vi "UI_Stop.vi"(0 "reference in":refnum<class "GUI.lvclass">, 5 "timeout ms":i32=1000, 11 "error in (no error)":errorcluster) -> (4 "reference out":refnum<class "GUI.lvclass">, 6 "timeout":bool, 10 "time":i32, 15 "error out":errorcluster)   [LabVIEW 2019, in "GUI.lvclass"]
uses:
  GUI.lvclass
  GUI.lvclass/GUI.ctl
  WindowsState.ctl
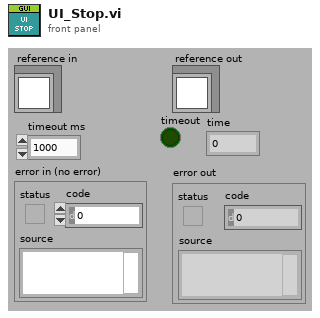
[diagram p1: front panel]
types:
  T1 = typedef "GUI.lvclass/WindowsState.ctl" = enum16{"NotReady", "Ready", "Inserted", "Opened"}
  T2 = typedef "GUI.lvclass/Shered Data.ctl" = cluster{"WindowsState":T1, "UI VI":refnum<vi>, "SubPnl":refnum<vi>}
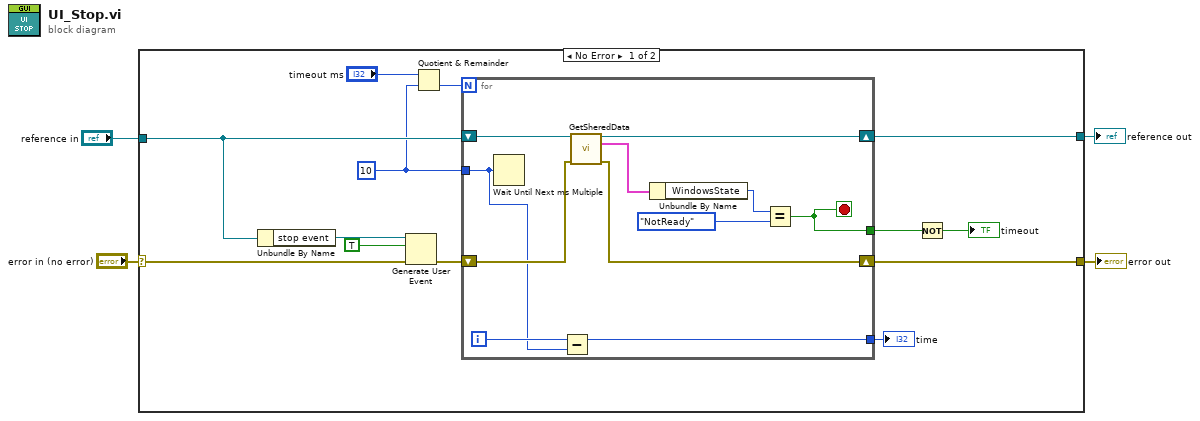
[diagram p0: block diagram]
diagram:
  n1 = case shown="No Error" "error in (no error)" {
    selector: "error in (no error)" -> [w17 w30]
    tunnel: [w10 w30] -> w3
    tunnel: [w11 w29] -> w1
    tunnel: "reference in" -> [w16 w29]
    frame No Error {
      w6 = u32 10 ("millisecond multiple")
      n2 = Unbundle By Name(w16) -> ("stop event"=w15:refnum<user-event>)
      n3 = Generate User Event(user event=w15, event data cluster=TRUE ("event data"), error in=w17) -> (error out=w12:errorcluster)  [unwired: 1 in, 1 out]
      n4 = Quotient & Remainder(x="timeout ms", y=w6) -> (floor(x/y)=w5:u32)  [unwired: 1 out]
      n5 = for {
        N: w5 -> [_]
        shift-right: [w24] -> w11
        shift-left: w16 -> [w25]
        shift-right: [w22] -> w10
        shift-left: w12 -> [w23]
        tunnel: [w27] -> w9
        tunnel: [w19] -> w7
        tunnel: w6 -> [w18]
        i -> [w26]
        stop <- w27 stop-if-true
        n6 = Wait Until Next ms Multiple(millisecond multiple=w18) -> ()  [unwired: 1 out]
        n7 = Subtract(x=w26, y=w18) -> (x-y=w19:u32)
        n8 = call "GetSheredData.vi"("reference in"=w25, "error in (no error)"=w23) -> ("reference out"=w24:refnum<class "GUI.lvclass">, "data"=w21:T2, "error out"=w22:errorcluster)  [unwired: 11 in]
        n9 = Unbundle By Name(w21) -> ("WindowsState"=w20:T1)
        n10 = Equal?(x=w20, y=WindowsState."NotReady") -> (x = y?=w27:bool)
      }
      "time" <- w7
      n11 = Not(x=w9) -> (.not. x?=→"timeout":bool)
    }
    frame Error {
    }
  }
  "error out" <- w3
  "reference out" <- w1
